vi "DAQmx Create Channel (AI-Strain-Rosette Strain Gage).vi"(0 "task in":refnum<k21>, 1 "maximum value":dbl=0.001 format="%0.7f", 2 "minimum value":dbl=-0.001 format="%0.7f", 5 "physical channels":tag, 7 "name to assign":string, 9 "rosette configuration":T1={"rosette type"=15968, "gage orientation"=0.0, "rosette measurements"=[15971]} {"rosette measurements" items=["Principal Strain 1"=15971, "Principal Strain 2"=15972, "Principal Strain Angle"=15973, "Cartesian Strain X"=15974, "Cartesian Strain Y"=15975, "Cartesian Shear Strain XY"=15976, "Maximum Shear Strain"=15977, "Maximum Shear Strain Angle"=15978]; "rosette type" items=["Rectangular Rosette"=15968, "Delta Rosette"=15969, "Tee Rosette"=15970]}, 11 "error in":errorcluster, 13 "bridge information":T2={"strain configuration"=10271, "lead wire resistance"=0.0, "voltage excitation source"=10200, "voltage excitation value"=2.5} {"voltage excitation source" items=["Internal"=10200, "External"=10167, "None"=10230]; "voltage excitation value" format="%0.2f"; "lead wire resistance" format="%0.2f"; "strain configuration" items=["Full Bridge I"=10183, "Full Bridge II"=10184, "Full Bridge III"=10185, "Half Bridge I"=10188, "Half Bridge II"=10189, "Quarter Bridge I"=10271, "Quarter Bridge II"=10272]}, 14 "strain gage information":T3={"gage factor"=2.0, "nominal gage resistance"=350.0, "poisson ratio"=0.3} {"poisson ratio" format="%0.2f"; "nominal gage resistance" format="%0.2f"; "gage factor" format="%0.2f"}) -> (4 "task out":refnum<k21>, 15 "error out":errorcluster)   [LabVIEW 2013]
doc: "Creates channels to measure two-dimensional strain using a rosette strain gage."
uses:
  C:/Program Files/National Instruments/LabVIEW 2013/resource/objmgr/daqmx.rc
panel:
  # "input limits"
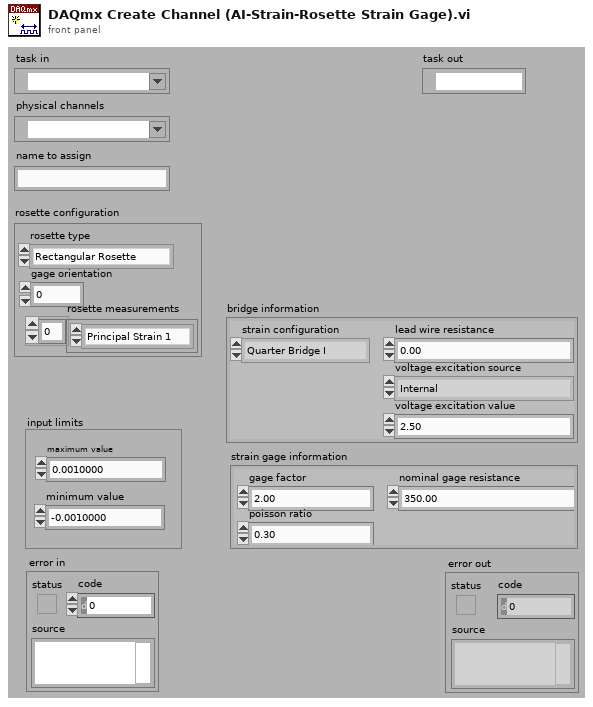
[diagram p1: front panel]
types:
  T1 = cluster{"rosette type":i32, "gage orientation":dbl, "rosette measurements":i32[]}
  T2 = cluster{"strain configuration":i32, "lead wire resistance":dbl, "voltage excitation source":i32, "voltage excitation value":dbl}
  T3 = cluster{"gage factor":dbl, "nominal gage resistance":dbl, "poisson ratio":dbl}
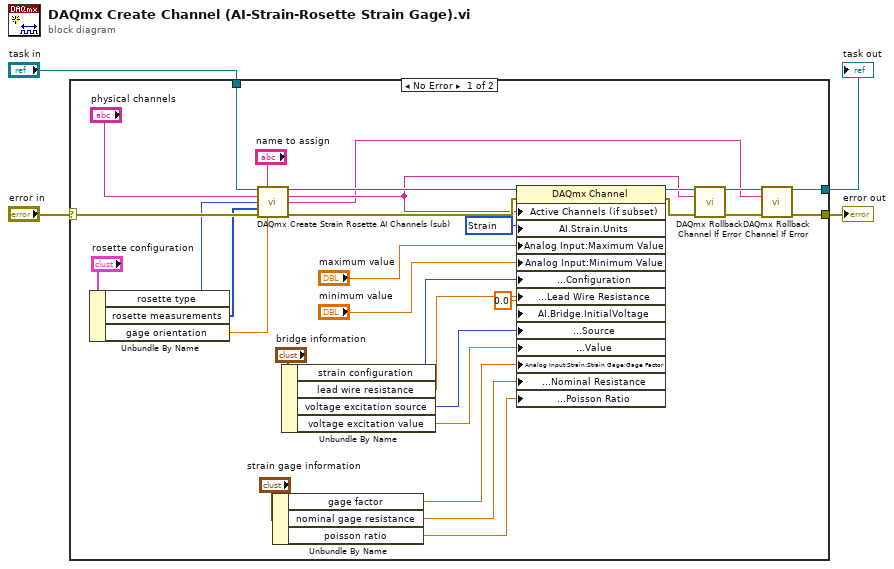
[diagram p0: block diagram]
diagram:
  n1 = case shown="No Error" "error in" {
    selector: "error in" -> [w34 w36]
    tunnel: [w12 w36] -> w4
    tunnel: "task in" -> [w35 w37]
    tunnel: [w13 w37] -> w1
    frame No Error {
      w6 = 10299 items=["Strain"=10299, "From Custom Scale"=10065] ("AI.Strain.Units")
      n2 = Unbundle By Name("rosette configuration") -> ("rosette type"=w9:i32, "rosette measurements"=w8:i32[], "gage orientation"=w7:dbl)
      n3 = call "DAQmx Create Strain Rosette AI Channels (sub).vi"("task in"=w35, "virtual channel name"="name to assign", "physical channel name"="physical channels", "rosette type"=w9, "rosette measurements"=w8, "error in"=w34, "gage orientation"=w7) -> ("task out"=w31:refnum<k21>, "raw strain channels"=w16:string, "calculated strain channels"=w11:string, "error out"=w28:errorcluster)  [unwired: 5 out]
      n4 = Unbundle By Name("strain gage information") -> ("gage factor"=w21:dbl, "nominal gage resistance"=w20:dbl, "poisson ratio"=w19:dbl)
      n5 = Unbundle By Name("bridge information") -> ("strain configuration"=w25:i32, "lead wire resistance"=w24:dbl, "voltage excitation source"=w23:i32, "voltage excitation value"=w22:dbl)
      n6 = property class="DAQmx Channel"(reference=w31, error in=w28, "Active Channels (if subset)"=w16, "AI.Strain.Units"=w6, "Analog Input:Maximum Value"="maximum value", "Analog Input:Minimum Value"="minimum value", "Analog Input:Strain:Strain Gage:Configuration"=w25, "Analog Input:General Properties:Signal Conditioning:Lead Wire Resistance"=w24, "AI.Bridge.InitialVoltage"=0.0, "Analog Input:General Properties:Signal Conditioning:Excitation:Source"=w23, "Analog Input:General Properties:Signal Conditioning:Excitation:Value"=w22, "Analog Input:Strain:Strain Gage:Gage Factor"=w21, "Analog Input:General Properties:Signal Conditioning:Bridge:Nominal Resistance"=w20, "Analog Input:Strain:Strain Gage:Poisson Ratio"=w19) -> (reference out=w18:refnum<k21>, error out=w17:errorcluster)
      n7 = call "DAQmx Rollback Channel If Error.vi"("task in"=w18, "channel names"=w16, "error in"=w17) -> ("task out"=w15:refnum<k21>, "error out"=w14:errorcluster)  [unwired: 11 out]
      n8 = call "DAQmx Rollback Channel If Error.vi"("task in"=w15, "channel names"=w11, "error in"=w14) -> ("task out"=w13:refnum<k21>, "error out"=w12:errorcluster)  [unwired: 11 out]
    }
    frame Error {
    }
  }
  "error out" <- w4
  "task out" <- w1
